vi "8.-Formula Node.vi"() -> ()   [LabVIEW 2020]
panel:
  out "Waveform Graph":dbl[](graph)
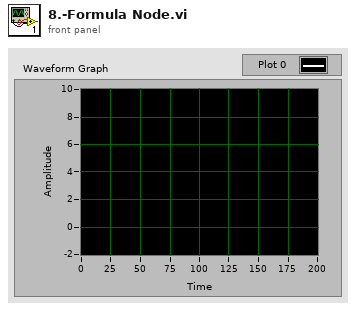
[diagram p1: front panel]
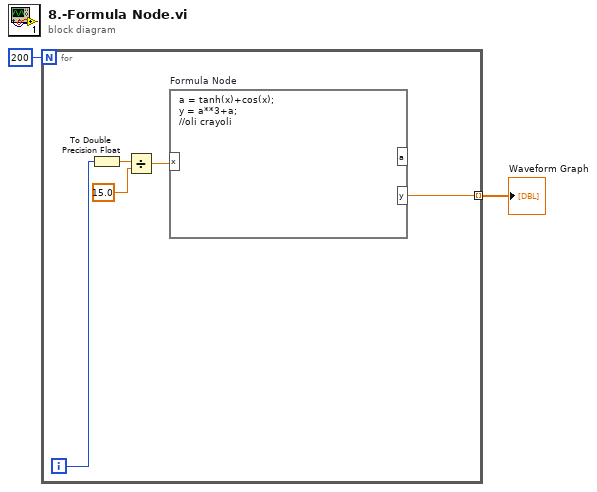
[diagram p0: block diagram]
diagram:
  n1 = for {
    N: 200 -> [_]
    tunnel: [w3] -> w1 mode=indexing
    i -> [w6]
    n2 = To Double Precision Float(number=w6) -> (double precision float=w7:dbl)
    n3 = Divide(x=w7, y=15.0) -> (x/y=w5:dbl)
    n4 = formula code="a = tanh(x)+cos(x);\ny = a**3+a;\n//oli crayoli"("x"=w5) -> ("y"=w3:dbl)  [unwired: 1 out]
  }
  "Waveform Graph" <- w1
